vi "Get Path to Transient Demo VI.vi"() -> (3 "Path to Transient Capture Subpanel":path)   [LabVIEW 2017]
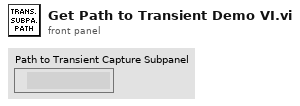
[diagram p1: front panel]
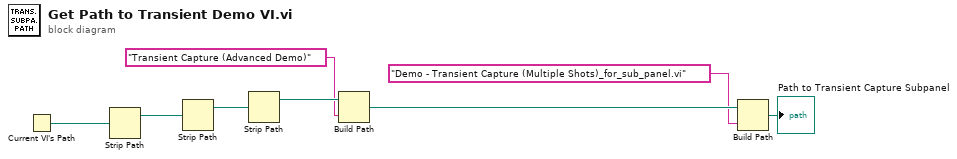
[diagram p0: block diagram]
diagram:
  n1 = Current VI's Path() -> (path=w8:path)
  n2 = Strip Path(path=w8) -> (stripped path=w7:path)  [unwired: 1 out]
  n3 = Strip Path(path=w7) -> (stripped path=w6:path)  [unwired: 1 out]
  n4 = Strip Path(path=w6) -> (stripped path=w5:path)  [unwired: 1 out]
  n5 = Build Path(base path=w5, name or relative path="Transient Capture (Advanced Demo)") -> (appended path=w3:path)
  n6 = Build Path(base path=w3, name or relative path="Demo - Transient Capture (Multiple Shots)_for_sub_panel.vi") -> (appended path=→"Path to Transient Capture Subpanel":path)
